vi "GV Nmax.vi"() -> ()   [LabVIEW 2017]
panel:
  out "Nmax":u32[](array[numeric])
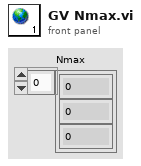
[diagram p1: front panel]
diagram:
